vi "convert_linear_pixel_index_to_coordinates.vi"(8 "error in (no error)":errorcluster, 10 "pixel indices":i32[](array[numeric]), 11 "Image in":refnum<class "Image.lvclass">) -> (0 "error out":errorcluster, 1 "y coordinates":i32[](array[numeric]), 2 "x coordinates":i32[](array[numeric]), 3 "Image out":refnum<class "Image.lvclass">)   [LabVIEW 2010, in "Image.lvclass"]
uses:
  Image.lvclass
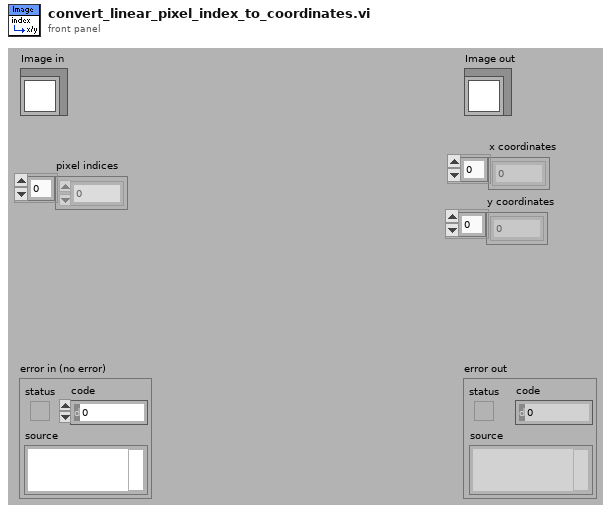
[diagram p1: front panel]
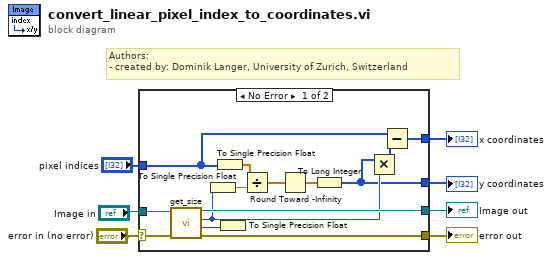
[diagram p0: block diagram]
diagram:
  # "Authors: \n- created by: Dominik Langer, University of Zurich, Switzerland"
  n1 = case shown="No Error" "error in (no error)" {
    selector: "error in (no error)" -> [w21 w23]
    tunnel: [w20 w23] -> w6
    tunnel: [w18 w22] -> w4
    tunnel: "Image in" -> [w19 w22]
    tunnel: "pixel indices" -> [w10 _]
    tunnel: [w11 _] -> w2
    tunnel: [w8 _] -> w1
    frame No Error {
      n2 = call-dynamic "get_size.vi"("error in (no error)"=w21, "Image in"=w19) -> ("error out"=w20:errorcluster, "y resolution"=w17:i32, "x resolution"=w12:i32, "Image out"=w18:refnum<class "Image.lvclass">)  [unwired: 2 in, 4 out]
      n3 = To Single Precision Float(number=w12) -> (single precision float=w15:sgl)
      n4 = To Single Precision Float(number=w10) -> (single precision float=w16:sgl[])
      n5 = To Single Precision Float(number=w17) -> ()  [unwired: 1 out]
      n6 = Divide(x=w16, y=w15) -> (x/y=w14:sgl[])
      n7 = Round Toward -Infinity(1:w14) -> (0:w13:sgl[])
      n8 = To Long Integer(number=w13) -> (32bit integer=w11:i32[])
      n9 = Multiply(x=w11, y=w12) -> (x*y=w9:i32[])
      n10 = Subtract(x=w10, y=w9) -> (x-y=w8:i32[])
    }
    frame Error {
    }
  }
  "error out" <- w6
  "Image out" <- w4
  "y coordinates" <- w2
  "x coordinates" <- w1
